vi "dvp Vi Set Accelerate Sel.vi"(10 "AccelerateSel":u32, 11 "handle":u32) -> (3 "function return":u32(ring))   [LabVIEW 2018, in "LabViewDVPCamera.lvlib"]
doc: "LabviewDvp2Api dvpStatus dvpViSetAccelerateSel(dvpHandle handle, dvpUint32 AccelerateSel);"
uses:
  LabViewDVPCamera.lvlib
  LabViewDVPCamera/LabViewDVPCamera.dll
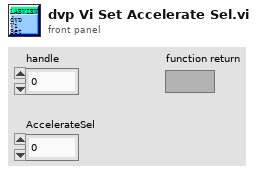
[diagram p1: front panel]
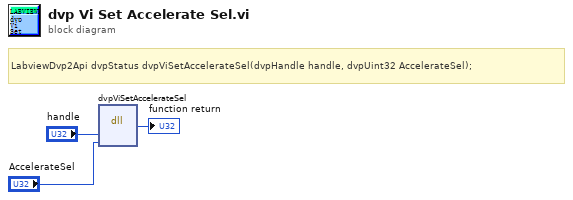
[diagram p0: block diagram]
diagram:
  # "LabviewDvp2Api dvpStatus dvpViSetAccelerateSel(dvpHandle handle, dvpUint32 AccelerateSel);"
  n1 = dll-call lib="C:/Program Files (x86)/DVP2 Labview cn 64/Sample/LabViewDVPCamera/LabViewDVPCamera.*" fn="dvpViSetAccelerateSel"("handle"="handle", "AccelerateSel"="AccelerateSel") -> (→"function return":u32)  [unwired: 5 in, 2 out]
